vi "FDMR script generator.vi"(9 "Generator options":T1, 10 "Prototype line":T2 {"Sampling Rate" items=["117 ks/S"=9, "58.6 kS/s"=10, "29.3 kS/s"=11, "14.6 kS/s"=12, "7.32 kS/s"=13, "3.66 kS/s"=14, "1.83 kS/s"=15]; "Angle [°]" min=-1.0 max=330.0; "ModA [G]" min=0.0 max=50.0; "Repeat [-]" min=0 max=1048576; "Points [-]" min=4096 max=5000000 step=1; "Field [T]" min=-16.0 max=16.0}, 11 "Editor script":T2[](array[typedef]) {"Sampling Rate" items=["117 ks/S"=9, "58.6 kS/s"=10, "29.3 kS/s"=11, "14.6 kS/s"=12, "7.32 kS/s"=13, "3.66 kS/s"=14, "1.83 kS/s"=15]; "Angle [°]" min=-1.0 max=330.0; "ModA [G]" min=0.0 max=50.0; "Repeat [-]" min=0 max=1048576; "Points [-]" min=4096 max=5000000 step=1; "Field [T]" min=-16.0 max=16.0}) -> (3 "Array":T2[](array[typedef]) {"Sampling Rate" items=["117 ks/S"=9, "58.6 kS/s"=10, "29.3 kS/s"=11, "14.6 kS/s"=12, "7.32 kS/s"=13, "3.66 kS/s"=14, "1.83 kS/s"=15]; "Angle [°]" min=-1.0 max=330.0; "ModA [G]" min=0.0 max=50.0; "Repeat [-]" min=0 max=1048576; "Points [-]" min=4096 max=5000000 step=1; "Field [T]" min=-16.0 max=16.0})   [LabVIEW 2024]
uses:
  Datatypes/FDMR+ script line.ctl
  Subsystem modules/Lock-in module/ctl/OSC sampling rate.ctl
  Datatypes/FDMR script generator options.ctl
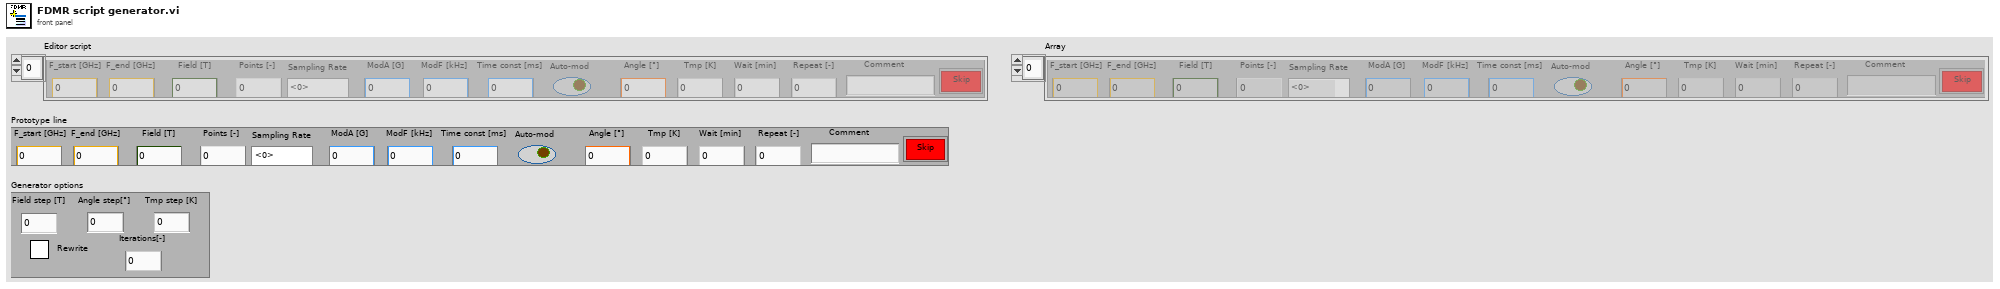
[diagram p1: front panel]
types:
  T1 = typedef "FDMR script generator options.ctl" = cluster{"Field step [T]":dbl, "Angle step[°]":dbl, "Tmp step [K]":dbl, "Iterations[-]":u16, "Script generator option":bool}
  T2 = typedef "FDMR+ script line.ctl" = cluster{"F_start [GHz]":dbl, "F_end [GHz]":dbl, "Field [T]":dbl, "Points [-]":u32, "Sampling Rate":T3, "ModA [G]":dbl, "ModF [kHz]":dbl, "Time const [ms]":dbl, "Angle [°]":dbl, "Tmp [K]":dbl, "Wait [min]":dbl, "Repeat [-]":i32, "Comment":string, "Execute":bool, "Auto-mod":bool}
  T3 = typedef "OSC sampling rate.ctl" = u16
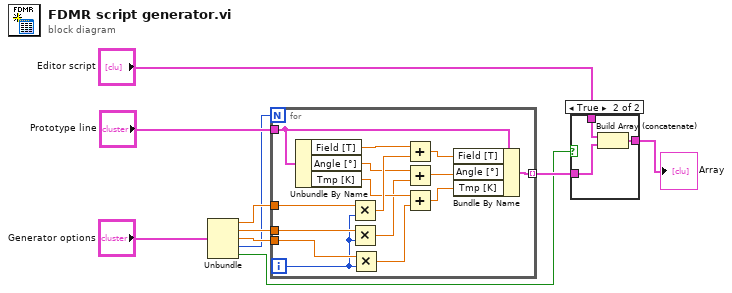
[diagram p0: block diagram]
diagram:
  n1 = Unbundle("Generator options") -> ("Field step [T]"=w8:dbl, "Angle step[°]"=w9:dbl, "Tmp step [K]"=w10:dbl, "Iterations[-]"=w6:u16, "Script generator option"=w1:bool)
  n2 = for {
    N: w6 -> [_]
    tunnel: "Prototype line" -> [w19]
    tunnel: w8 -> [w25]
    tunnel: w9 -> [w24]
    tunnel: w10 -> [w23]
    tunnel: [w11] -> w3 mode=indexing
    i -> [w22]
    n3 = Unbundle By Name(w19) -> ("Field [T]"=w18:dbl, "Angle [°]"=w17:dbl, "Tmp [K]"=w16:dbl)
    n4 = Multiply(x=w25, y=w22) -> (x*y=w20:dbl)
    n5 = Multiply(x=w24, y=w22) -> (x*y=w12:dbl)
    n6 = Multiply(x=w23, y=w22) -> (x*y=w21:dbl)
    n7 = Add(x=w18, y=w20) -> (x+y=w15:dbl)
    n8 = Add(x=w17, y=w12) -> (x+y=w14:dbl)
    n9 = Add(x=w16, y=w21) -> (x+y=w13:dbl)
    n10 = Bundle By Name(cluster=w19, "Field [T]"=w15, "Angle [°]"=w14, "Tmp [K]"=w13) -> (w11:T2)
  }
  n11 = case shown="True" w1 {
    tunnel: "Editor script" -> [_ w29]
    tunnel: w3 -> [w26 w28]
    tunnel: [w26 w27] -> w2
    frame False {
    }
    frame True {
      n12 = Build Array (concatenate)(w29, w28) -> (w27:T2[])
    }
  }
  "Array" <- w2
